vi "Write  Swich Rule and Polarity.vi"(0 "class data in":refnum<class "MB_ENGINE.lvclass">, 5 "SW":u16, 7 "Switch Rule and Polarity":T1, 11 "error in (no error)":errorcluster) -> (4 "class data out":refnum<class "MB_ENGINE.lvclass">, 15 "error out":errorcluster)   [LabVIEW 2019, in "MB_ENGINE.lvclass"]
uses:
  MB_ENGINE.lvclass
  Switch Rule and Polarity.ctl
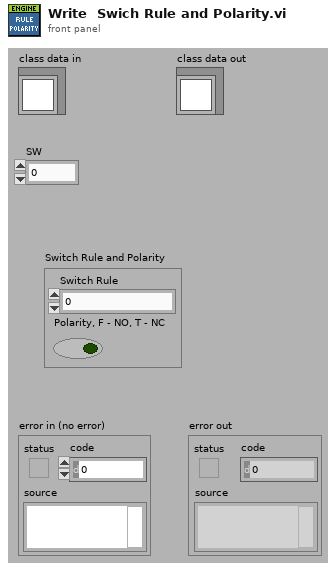
[diagram p1: front panel]
types:
  T1 = typedef "MB_ENGINE.lvclass/Switch Rule and Polarity.ctl" = cluster{"Switch Rule":u8, "Polarity, F - NO, T - NC":bool}
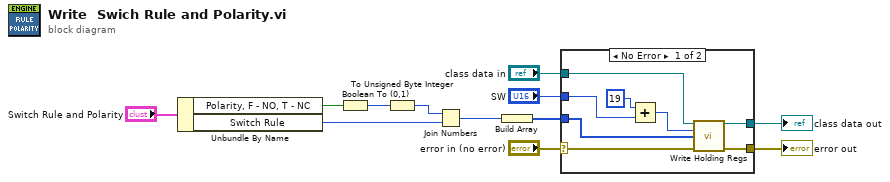
[diagram p0: block diagram]
diagram:
  n1 = Unbundle By Name("Switch Rule and Polarity") -> ("Polarity, F - NO, T - NC"=w4:bool, "Switch Rule"=w6:u8)
  n2 = Boolean To (0,1)(Boolean=w4) -> (0, 1=w3:i16)
  n3 = To Unsigned Byte Integer(number=w3) -> (unsigned 8bit integer=w5:u8)
  n4 = Join Numbers(hi=w5, lo=w6) -> ((hi.lo)=w2:u16)
  n5 = Build Array(w2) -> (w1:u16[])
  n6 = case shown="No Error" "error in (no error)" {
    selector: "error in (no error)" -> [w19 w22]
    tunnel: [w17 w22] -> w11
    tunnel: "class data in" -> [w20 w21]
    tunnel: [w13 w21] -> w9
    tunnel: "SW" -> [w15 _]
    tunnel: w1 -> [w14 _]
    frame No Error {
      n7 = Add(x=u16 19 ("starting address"), y=w15) -> (x+y=w16:u16)
      n8 = call-dynamic "Write Holding Regs.vi"("reference in"=w20, "starting address"=w16, "Regs"=w14, "error in (no error)"=w19) -> ("reference out"=w13:refnum<class "MB_ENGINE.lvclass">, "error out"=w17:errorcluster)  [unwired: 10 in]
    }
    frame Error {
    }
  }
  "error out" <- w11
  "class data out" <- w9
